vi "Eyeblinker-Go.vi"(7 "Device reference":refnum<vi>, 8 "error in (no error)":errorcluster) -> (0 "error out":errorcluster)   [LabVIEW 2015]
doc: "Pulses a juicer valve.\n\nDevice reference: which valve?\nDuration: how long to open for?\n--positive: specifies open duration in ms\n--unwired or 0: accept default from valve ref.\n--negative: open indefinitely\nEventstring: used for timestamping\n--empty: no timestamp will be generated\n--unwired or \"auto-generate\": TS w/ default eventstring\n--otherwise: TS with user-provided string\nAcutal duration: the actual commanded pulse duration. Useful if you decided to use the default value.\n\nThe default eventstring is:\n[valve name].open.[duration]\nwhere [valve name] is the referenced valve's front panel label text and [duration] will have the actual duration filled in if the Duration input was left unwired (or set to 0)."
uses:
  Typedefs/Eyeblinker.ctl
  Rack/Typedefs/OutputRequest refnum.ctl
  Rack/Typedefs/OutputRequest.ctl
  Rack/Typedefs/InputData cluster.ctl
  Rack/Methods/Port drivers/DigitalInput-DataCluster.ctl
panel:
  # "(must be on same NI card)"
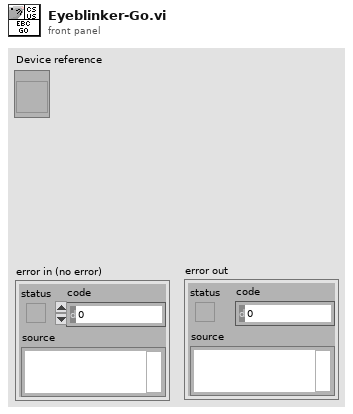
[diagram p1: front panel]
types:
  T1 = typedef "Eyeblinker.ctl" = cluster{"Settings":cluster{"Timestamp port name":string, "Port name":string, "Port index":i32}, "OutputRequest event ref":T2, "InputData reference":refnum<vi>}
  T2 = typedef "OutputRequest refnum.ctl" = refnum<user-event>
  T3 = typedef "OutputRequest.ctl" = cluster{"Target":string, "Command":string}
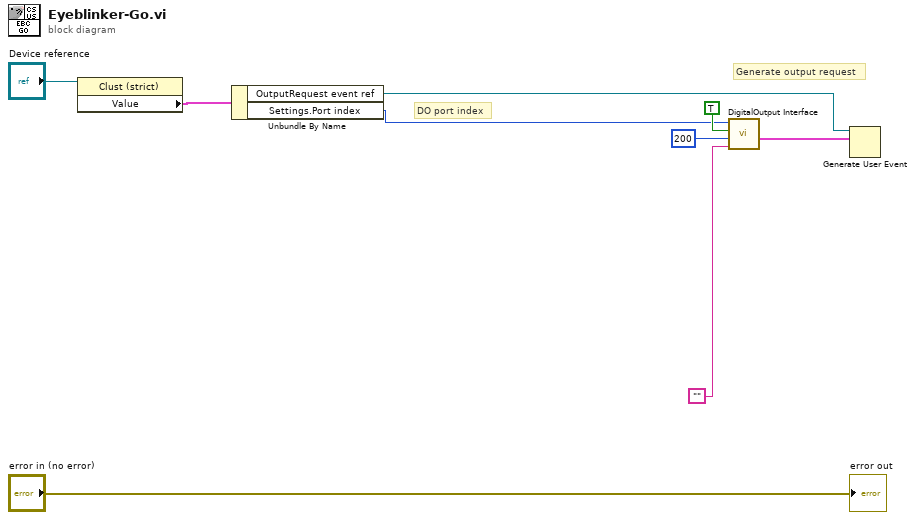
[diagram p0: block diagram]
diagram:
  # "DO port index"
  # "Generate output request"
  n1 = property class="Clust (strict)"(reference="Device reference") -> ("Value"=w9:T1)  [unwired: 1 in, 2 out]
  n2 = Unbundle By Name(w9) -> ("OutputRequest event ref"=w5:T2, "Settings.Port index"=w3:i32)
  n3 = call "DigitalOutput Interface.vi"("Eventstring"="", "Pulse duration (-1 for cont.)"=200, "On/off"=TRUE, "Port index"=w3) -> ("OutputRequest"=w6:T3)  [unwired: 7 in]
  n4 = Generate User Event(user event=w5, event data cluster=w6) -> ()  [unwired: 2 in, 2 out]
  "error out" <- "error in (no error)"
